vi "readSDOU16.vi"(6 "subIndex":u8, 8 "error in (no error)":errorcluster, 9 "objectIndex":u16 format="%x", 10 "interface object in":refnum<k20>, 11 "MotorController in":refnum<class "MotorController.lvclass">) -> (0 "error out":errorcluster, 1 "output":u16, 2 "interface object out":refnum<k20>, 3 "MotorController out":refnum<class "MotorController.lvclass">)   [LabVIEW 2018, in "MotorController.lvclass"]
uses:
  MotorController.lvclass
  MotorController.lvclass/MotorController.ctl
  <vilib>/CANopenLib/CANOPEN.llb/CANopen SDO Create.vi
  <vilib>/CANopenLib/CANOPEN.llb/CANopen SDO Read [U16].vi
  <vilib>/CANopenLib/CANOPEN.llb/CANopen SDO Close.vi
panel:
  out "completion code":u32 format="%.0x"
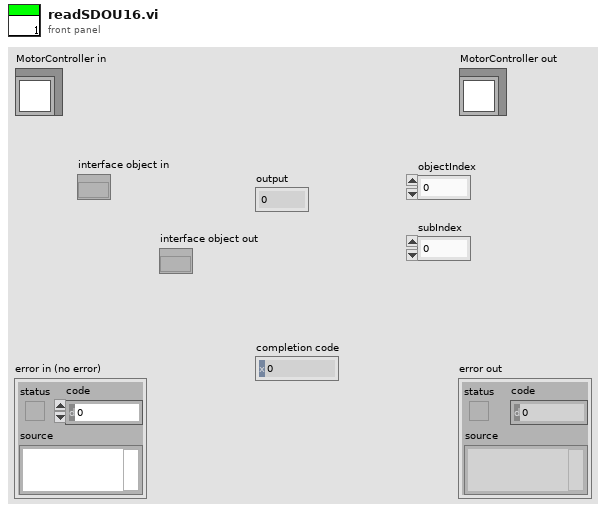
[diagram p1: front panel]
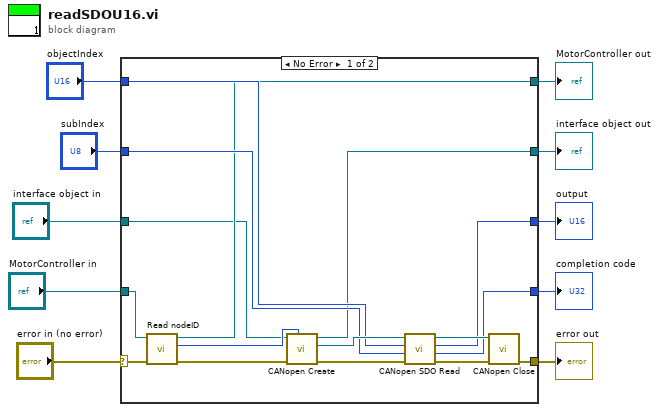
[diagram p0: block diagram]
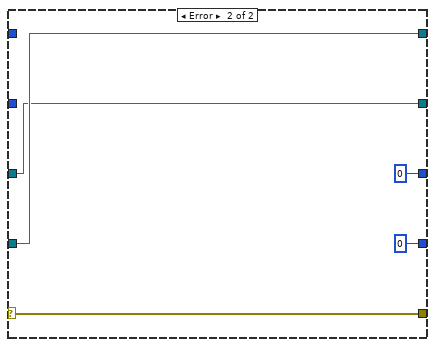
[diagram p2: hidden frame]
diagram:
  n1 = case shown="No Error" "error in (no error)" {
    selector: "error in (no error)" -> [w16 w31]
    tunnel: [w14 w31] -> w3
    tunnel: [w18 w30] -> w2
    tunnel: "MotorController in" -> [w17 w30]
    tunnel: "subIndex" -> [w20 _]
    tunnel: "objectIndex" -> [w19 _]
    tunnel: "interface object in" -> [w15 w29]
    tunnel: [w13 w29] -> w7
    tunnel: [w12 u32 0 ("completion code")] -> w6
    tunnel: [w11 u16 0 ("U16 data")] -> w1
    frame No Error {
      n2 = call "Read nodeID.vi"("error in (no error)"=w16, "MotorController in"=w17) -> ("error out"=w25:errorcluster, "nodeID"=w26:u8, "MotorController out"=w18:refnum<class "MotorController.lvclass">)  [unwired: 7 in]
      n3 = call-poly <vilib>:"CANopen Create.vi"("node-ID"=w26, "error in (no error)"=w25, "interface object in"=w15) -> ("error out"=w24:errorcluster, "SDO object out"=w23:refnum<k20>, "interface object out"=w13:refnum<k20>)  [unwired: 6 in]
      n4 = call-poly <vilib>:"CANopen SDO Read.vi"("error in (no error)"=w24, "object sub-index (0)"=w20, "object index"=w19, "SDO object in"=w23) -> ("error out"=w21:errorcluster, "completion code"=w12:u32, "U16 data"=w11:u16, "SDO object out"=w22:refnum<k20>)  [unwired: 4 in]
      n5 = call-poly <vilib>:"CANopen Close.vi"("error in (no error)"=w21, "SDO object in"=w22) -> ("error out"=w14:errorcluster)  [unwired: 9 in]
    }
    frame Error {
    }
  }
  "error out" <- w3
  "MotorController out" <- w2
  "output" <- w1
  "interface object out" <- w7
  "completion code" <- w6
